vi "Camera_CheckCameraSetting.vi"(11 "CameraName":refnum<vi>) -> (2 "CameraGot?":bool, 3 "Camera Session":T1)   [LabVIEW 2019]
uses:
  <vilib>/userdefined/High Color/IMAQdx.ctl
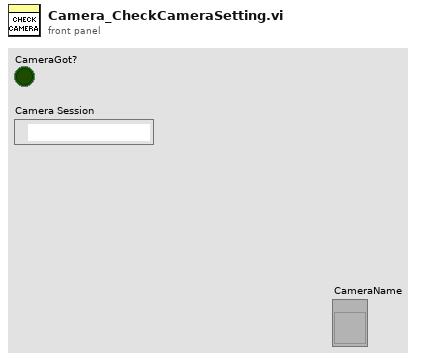
[diagram p1: front panel]
types:
  T1 = typedef "IMAQdx.ctl" = refnum<k21>
  T2 = enum16{"Init", "Grab", "Get All", "Close", "Set Camera"}
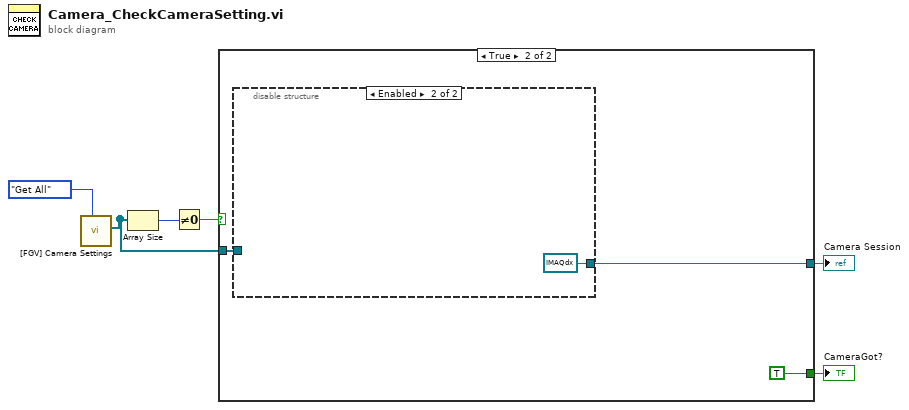
[diagram p0: block diagram]
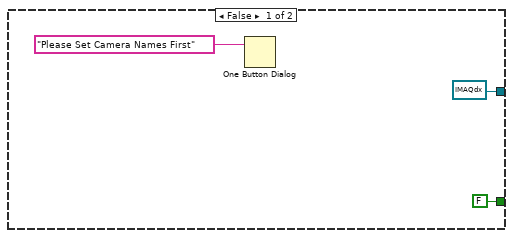
[diagram p2: hidden frame]
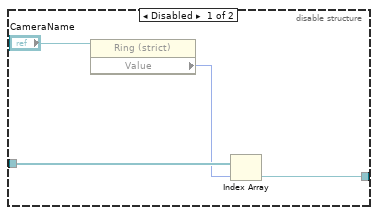
[diagram p3: hidden frame]
diagram:
  n1 = call "[FGV] Camera Settings.vi"("Action"=T2."Get All") -> ("Camera Interface Name"=w1:T1[])  [unwired: 8 in, 2 out]
  n2 = Array Size(array=w1) -> (size(s)=w6:i32)
  n3 = Not Equal To 0?(x=w6) -> (x != 0?=w5:bool)
  n4 = case shown="True" w5 {
    tunnel: [FALSE TRUE] -> w4
    tunnel: w1 -> [_ w11]
    tunnel: [T1 refnum ("Camera Session") w10] -> w3
    frame False {
      n5 = One Button Dialog(message="Please Set Camera Names First") -> ()  [unwired: 1 in, 1 out]
    }
    frame True {
      n6 = disable-structure shown="Enabled" {
        disable-tunnel: w11 -> [w15 _]
        disable-tunnel: [w13 T1 refnum ("Session Out")] -> w10
        frame Disabled {
          n7 = property class="Ring (strict)"(reference="CameraName") -> ("Value"=w14:u16)  [unwired: 1 in, 2 out]
          n8 = Index Array(array=w15, index=w14) -> (element=w13:T1)
        }
        frame Enabled {
        }
      }
    }
  }
  "CameraGot?" <- w4
  "Camera Session" <- w3
